vi "Align using camera.vi"(1 "X":dbl format="%.2f", 2 "Enable?":bool, 3 "setpoint":dbl format="%.2f") -> (0 "X Output":dbl format="%.2f")   [LabVIEW 2013]
uses:
  <vilib>/addons/control/pid/pid.llb/PID (DBL).vi
  <vilib>/addons/control/pid/NI_PID_pid.lvlib
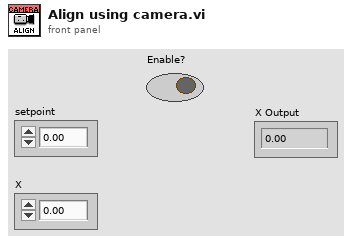
[diagram p1: front panel]
types:
  T1 = cluster{"proportional gain (Kc)":dbl, "integral time (Ti, min)":dbl, "derivative time (Td, min)":dbl}
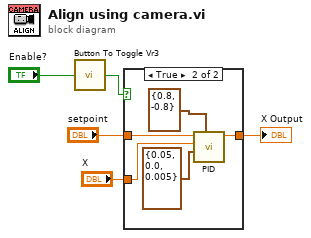
[diagram p0: block diagram]
diagram:
  n1 = call "Button To Toggle Vr3.vi"("InValue"="Enable?") -> ("Result"=w3:bool)
  n2 = case shown="True" w3 {
    tunnel: [w6 w9] -> w5
    tunnel: "setpoint" -> [_ w8]
    tunnel: "X" -> [w6 w7]
    frame False {
    }
    frame True {
      n3 = call-poly <vilib>:"PID.vi"("output range"=cluster{"output high":dbl, "output low":dbl} {"output high"=0.8, "output low"=-0.8}, "PID gains"=T1 {"proportional gain (Kc)"=0.05, "integral time (Ti, min)"=0.0, "derivative time (Td, min)"=0.005}, "process variable"=w7, "setpoint"=w8) -> ("output"=w9:dbl)  [unwired: 6 in, 1 out]
    }
  }
  "X Output" <- w5
